vi "KBRD Far (SubVI).vi"(11 "Queue in":refnum<queue>) -> ()   [LabVIEW 2018]
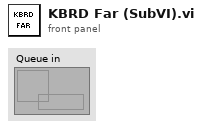
[diagram p1: front panel]
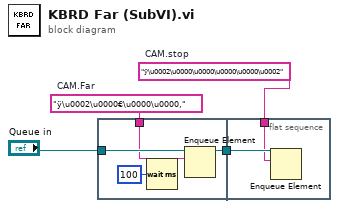
[diagram p0: block diagram]
diagram:
  w3 = "ÿ\u0002\u0000\u0000\u0000\u0000\u0002"  # CAM.stop
  w2 = "ÿ\u0002\u0000€\u0000\u0000‚"  # CAM.Far
  n1 = flat-sequence {
    tunnel: "Queue in" -> [w7]
    tunnel: w2 -> [w6]
    tunnel: [w5] -> w4
    tunnel: w4 -> [w10]
    tunnel: w3 -> [w9]
    frame #0 {
      n2 = Wait (ms)(milliseconds to wait=u32 100) -> ()  [unwired: 1 out]
      n3 = Enqueue Element(queue=w7, element=w6) -> (queue out=w5:refnum<queue>)  [unwired: 2 in, 2 out]
    }
    frame #1 {
      n4 = Enqueue Element(queue=w10, element=w9) -> ()  [unwired: 2 in, 3 out]
    }
  }
